vi "VI to C code.vi"() -> ()   [LabVIEW 2014, in "LabVIEW Universal Transcriptor SD Card Library.lvlib"]
uses:
  LabVIEW Universal Transcriptor SD Card Library.lvlib
panel:
  out "transcripted code":string
  in  "vi path":path=path "C:/Users/lubo/Documents/LabView/LabVIEW-Universal-Transcriptor-SD-Card-Library/Examples/listfiles.vi"
  in  "Includes":string[](array[string])=["<vector>"]
  in  "Defines":string[](array[string])=["using namespace std;"]
  out "error out":errorcluster
  in  "error in":errorcluster
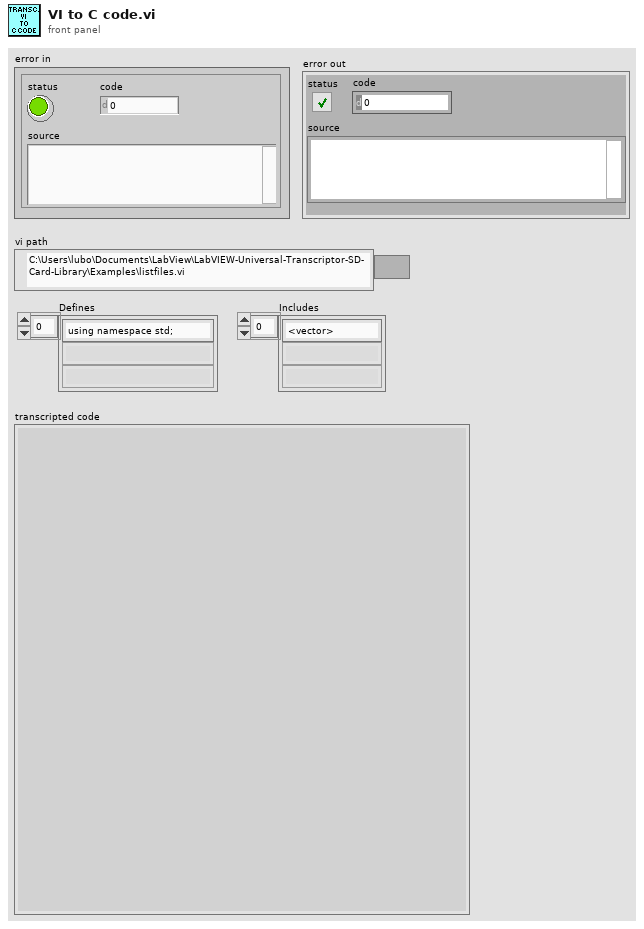
[diagram p1: front panel]
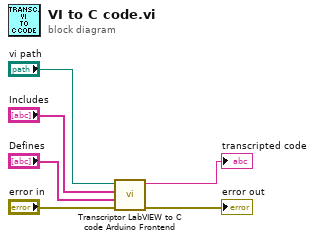
[diagram p0: block diagram]
diagram:
  n1 = call <vilib>:"Transcriptor LabVIEW to C code Arduino Frontend.vi"("error in"="error in", "Defines"="Defines", "Includes"="Includes", "vi path"="vi path") -> ("error out"=→"error out":errorcluster, "transcripted code"=→"transcripted code":string)  [unwired: 6 in]
